vi "ex2  structure condition.vi"() -> ()   [LabVIEW 2019]
panel:
  in  "number":dbl
  out "square root value":dbl
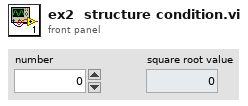
[diagram p1: front panel]
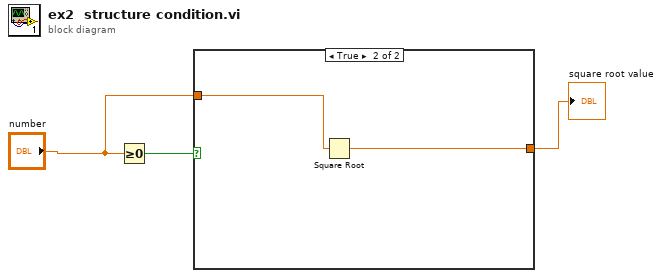
[diagram p0: block diagram]
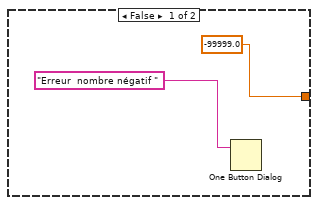
[diagram p2: hidden frame]
diagram:
  n1 = Greater Or Equal To 0?(x="number") -> (x >= 0?=w2:bool)
  n2 = case shown="True" w2 {
    tunnel: [-99999.0 ("valeur invalide") w6] -> w3
    tunnel: "number" -> [_ w7]
    frame False {
      n3 = One Button Dialog(message="Erreur  nombre négatif " ("String")) -> ()  [unwired: 1 in, 1 out]
    }
    frame True {
      n4 = Square Root(x=w7) -> (sqrt(x)=w6:dbl)
    }
  }
  "square root value" <- w3
